vi "Intake Loop.vi"   [LabVIEW 2017]
uses:
  <vilib>/Rock Robotics/WPI/ThirdParty/Phoenix-LabVIEW/Motor Controller/Controls/CTRE_Phoenix_MotorControl_ControlMode.ctl
  <vilib>/Rock Robotics/WPI/ThirdParty/Phoenix-LabVIEW/Motor Controller/Get/CTRE_Phoenix_MotorController_GetSelectedSensorData.vi
  <vilib>/Rock Robotics/WPI/ThirdParty/Phoenix-LabVIEW/Motor Controller/Get/CTRE_Phoenix_MotorController_GetOutputCurrent_Enhanced.vi
  <vilib>/Rock Robotics/WPI/ThirdParty/Phoenix-LabVIEW/Motor Controller/Get/CTRE_Phoenix_MotorController_GetPulseWidthAll.vi
  <vilib>/Rock Robotics/WPI/ThirdParty/Phoenix-LabVIEW/Motor Controller/Get/CTRE_Phoenix_MotorController_GetVoltage.vi
  <vilib>/Rock Robotics/WPI/ThirdParty/Phoenix-LabVIEW/Motor Controller/Get/CTRE_Phoenix_MotorController_GetGeneralStatus.vi
  <vilib>/Rock Robotics/WPI/ThirdParty/Phoenix-LabVIEW/Motor Controller/Get/CTRE_Phoenix_MotorController_GetTemperature.vi
  Robot Global Data.vi
  <vilib>/Rock Robotics/WPI/Solenoid/Deprecated/WPI_SolenoidSetBool.vi
types:
  T1 = typedef "CTRE_Phoenix_MotorControl_ControlMode.ctl" = u16
  T2 = typedef "Intake Status Cluster.ctl" = cluster{"Intake Mode":T3, "Intake States":T4, "Intake Current Angle":dbl, "Cube In Posession?":bool, "Intake Wrist Up?":bool}
  T3 = typedef "Intake Mode.ctl" = enum16{"Auto", "Semi Auto", "Manual"}
  T4 = typedef "Intake States.ctl" = enum16{"Zero", "Override Angle", "Idle", "Drop Mid", "Drop Low", "Outtake", "Intake"}
  T5 = typedef "Intake Command Cluster.ctl" = cluster{"Intake Mode":T3, "Intake States":T4, "Manual Roller Power":dbl, "Manual Close?":bool, "Manual Lift Power":dbl, "Override Lift?":bool, "Override Angle":dbl}
  T6 = typedef "Dashboard Control Data.ctl" = cluster{"Drivetrain Settings Cluster":T7, "Intake Presets":T9, "Elevator Settings Cluster":T10}
  T7 = typedef "Drivetrain Settings Cluster.ctl" = cluster{"Gyro Steer PID Gains":T8, "Distance Drive PID Gains":T8, "Drive Tolerance":dbl, "Gyro Tolerance":dbl, "Gyro Output":dbl, "Distance Output":dbl, "Y Power Multiplier":dbl, "Turn Power Multiplier":dbl, "Creep Rate":dbl, "Constant Power":bool, "DT Mode Modifier":enum16{"None, Default", "Cube", "Square"}, "Left Encoder Tick Constant":dbl, "Right Encoder Tick Constant":dbl, "Shift Speed":dbl}
  T8 = typedef "PID Gains Cluster.ctl" = cluster{"Integral Time":dbl, "Proportional Gain":dbl, "Derivative Time":dbl}
  T9 = typedef "Intake Presets.ctl" = cluster{"Idle Angle":dbl, "Mid Angle":dbl, "Low Angle":dbl, "Outtake Power":dbl, "Intake Power":dbl, "Unstuck":dbl, "Angle Tolerance":dbl, "Max Angle":dbl, "Max Current":dbl, "Current Trip Time":dbl, "Reset Encoder?":bool, "Encoder Scale":dbl, "PID gains":cluster{"proportional gain (Kc)":dbl, "integral time (Ti, min)":dbl, "derivative time (Td, min)":dbl}, "output range":cluster{"output high":dbl, "output low":dbl}}
  T10 = typedef "Elevator Settings Cluster.ctl" = cluster{"Ground Height":dbl, "Switch Height":dbl, "Scale High Height ":dbl, "Scale Low Height":dbl, "Elevator PID Gains":T11, "Elevator Tolerance":dbl, "Reset Encoders":bool, "Encoder Scale":dbl, "Max Height":dbl, "Mid Height":dbl, "output range":cluster{"output high":dbl, "output low":dbl}}
  T11 = typedef "PID Gains.ctl" = cluster{"proportional gain (Kc)":dbl, "integral time (Ti, min)":dbl, "derivative time (Td, min)":dbl}
  T12 = typedef "WPI_MotorControlDeviceRef.ctl" = cluster{"DeviceStatus":errorcluster, "Type":T13, "PWM":cluster{"PWM Channel":T14, "DeadBand":T15}, "CAN":cluster{"Device Number":u8, "SetOutput VI Ref":variant, "GetOutput VI Ref":variant, "Enable VI Ref":variant, "Disable VI Ref":variant, "Data":variant}, "Invert":bool, "DIO PWM":cluster{"PWM \"Enable\" Channel":T14, "DIOChannel":T16, "PWM Rate":dbl}}
  T13 = typedef "WPI_MotorControlType.ctl" = enum16{"PWM", "CAN", "DIO PWM"}
  T14 = typedef "FPGA_DIOPWMChannel.ctl" = enum8{"PWM 0", "PWM 1", "PWM 2", "PWM 3", "PWM 4", "PWM 5", "PWM 6", "PWM 7", "PWM 8", "PWM 9", "PWM MXP 0", "PWM MXP 1", "PWM MXP 2", "PWM MXP 3", "PWM MXP 4", "PWM MXP 5", "PWM MXP 6", "PWM MXP 7", "PWM MXP 8", "PWM MXP 9", "Invalid"}
  T15 = typedef "WPI_PWMDeadband.ctl" = cluster{"Name":string, "maxPositivePwm":i32, "minPositivePwm":i32, "centerPwm":i32, "maxNegativePwm":i32, "minNegativePwm":i32, "angularRange":u16}
  T16 = typedef "FPGA_DIOChannel.ctl" = enum8{"DIO 0", "DIO 1", "DIO 2", "DIO 3", "DIO 4", "DIO 5", "DIO 6", "DIO 7", "DIO 8", "DIO 9", "DIO MXP 0", "DIO MXP 1", "DIO MXP 2", "DIO MXP 3", "DIO MXP 4", "DIO MXP 5", "DIO MXP 6", "DIO MXP 7", "DIO MXP 8", "DIO MXP 9", "DIO MXP 10", "DIO MXP 11", "DIO MXP 12", "DIO MXP 13", "DIO MXP 14", "DIO MXP 15", "SPI Port CS1", "SPI Port CS2", "SPI Port CS3", "SPI Port MISO", "SPI Port MOSI", "Invalid"}
  T17 = typedef "WPI_SwitchDevRef.ctl" = cluster{"DevStatus":errorcluster, "DIO Channel":T16, "CntIndex":T18, "Normally Closed":bool}
  T18 = typedef "FPGA_CounterCtrSystemIndex.ctl" = enum8{"Ctr 0", "Ctr 1", "Ctr 2", "Ctr 3", "Ctr 4", "Ctr 5", "Ctr 6", "Ctr 7", "Invalid"}
  T19 = typedef "WPI_SolenoidDevRef.ctl" = cluster{"DevStatus":errorcluster, "Pneumatics Control Module":u8, "Forward Solenoid Channel":T20, "Reverse Solenoid Channel":T20}
  T20 = typedef "WPI_SolenoidChannel.ctl" = enum8{"Solenoid 0", "Solenoid 1", "Solenoid 2", "Solenoid 3", "Solenoid 4", "Solenoid 5", "Solenoid 6", "Solenoid 7", "Invalid"}
  T21 = typedef "Intake PDP Info.ctl" = cluster{"Voltage Percent Output":dbl, "Output Voltage":dbl, "Bus Voltage":dbl, "Device ID":dbl, "Output Current":dbl, "Sensor Velocity":dbl, "Sensor Position":dbl, "Pulse Width Position":dbl, "Pulse Width Velocity":dbl, "Temperature":dbl, "Inverted?":bool}
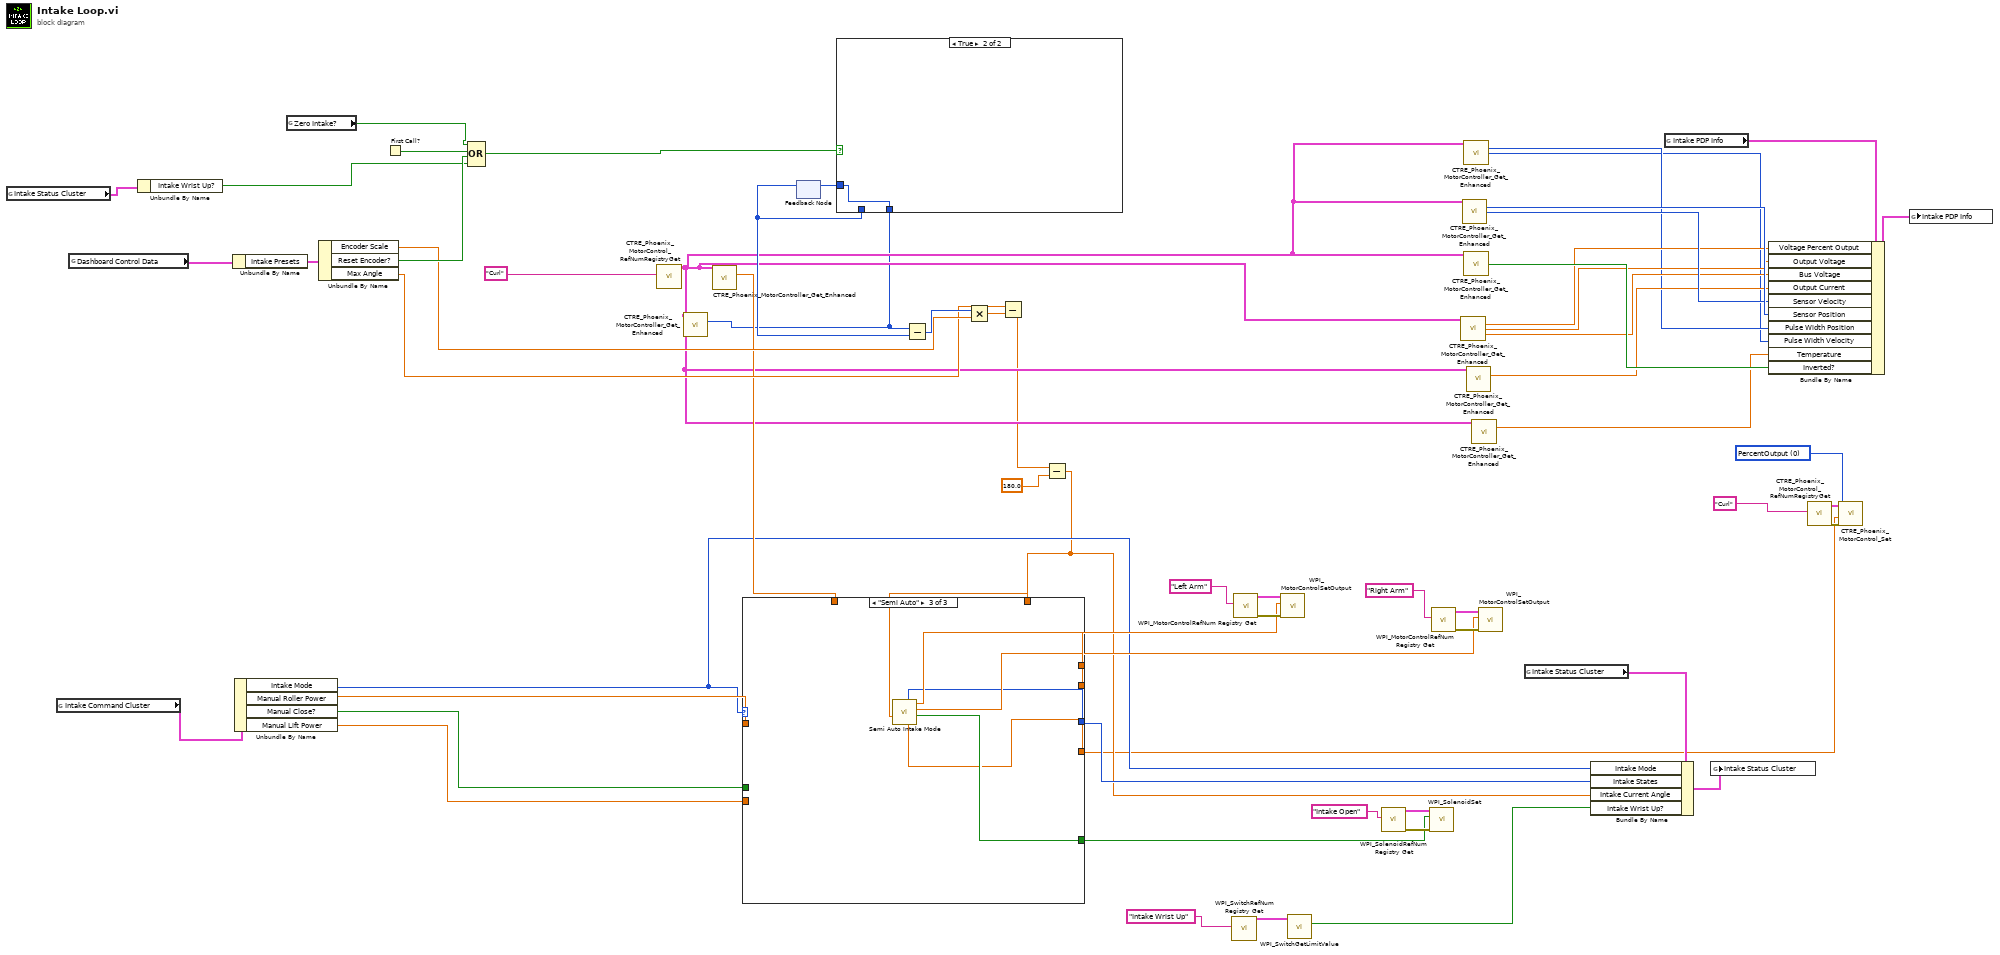
[diagram p0: block diagram]
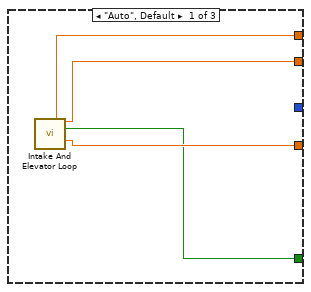
[diagram p2: hidden frame]
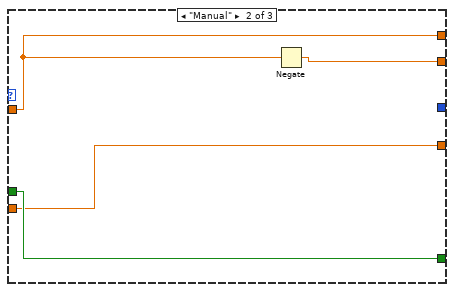
[diagram p3: hidden frame]
diagram:
  w25 = T1 0 items=["PercentOutput"=0, "Position"=1, "Velocity"=2, "Current"=3, "Follower"=5, "MotionProfile"=6, "MotionMagic"=7, "MotionMagicArc"=8, "MotionProfileArc"=10, "Disabled"=15] ("Control Mode")
  n1 = global read "Robot Global Data.vi" "Intake Status Cluster"() -> (w4:T2)
  n2 = global read "Robot Global Data.vi" "Intake Command Cluster"() -> (w52:T5)
  n3 = global read "Robot Global Data.vi" "Dashboard Control Data"() -> (w51:T6)
  n4 = Unbundle By Name(w4) -> ("Intake Wrist Up?"=w3:bool)
  n5 = Unbundle By Name(w51) -> ("Intake Presets"=w50:T9)
  n6 = Unbundle By Name(w52) -> ("Intake Mode"=w10:T3, "Manual Roller Power"=w34:dbl, "Manual Close?"=w33:bool, "Manual Lift Power"=w32:dbl)
  n7 = global read "Robot Global Data.vi" "Zero Intake?"() -> (w47:bool)
  n8 = Unbundle By Name(w50) -> ("Encoder Scale"=w42:dbl, "Reset Encoder?"=w48:bool, "Max Angle"=w40:dbl)
  n9 = First Call?() -> (First Call?: T/F=w49:bool)
  n10 = Compound Arithmetic op=OR(w47, w49, w48, w3) -> (w46:bool)
  n11 = call <vilib>:"CTRE_Phoenix_MotorControl_RefNumRegistryGet.vi"("refnum name"="Curl") -> ("PhoenixMotorControlDevRef"=w19:T12)  [unwired: 9 in, 1 out]
  n12 = call-poly <vilib>:"CTRE_Phoenix_MotorController_Get_Enhanced.vi"("PhoenixMotorControlDevRef"=w19) -> ("Position (Raw Sensor Units)"=w18:i32)  [unwired: 11 in, 3 out]
  n13 = call-poly <vilib>:"CTRE_Phoenix_MotorController_Get_Enhanced.vi"("PhoenixMotorControlDevRef"=w19) -> ("Output Current"=w20:dbl)  [unwired: 12 in, 2 out]
  n14 = feedback #1() -> (w44:i32)  [unwired: 1 in]
  n15 = case shown="True" w46 {
    tunnel: [w62 w63] -> w45
    tunnel: w44 -> [w62 _]
    tunnel: w18 -> [_ w63]
    frame False {
    }
    frame True {
    }
  }
  n16 = feedback-in #1(w45) -> ()
  n17 = Subtract(x=w18, y=w44) -> (x-y=w43:i32)
  n18 = Multiply(x=w43, y=w42) -> (x*y=w41:dbl)
  n19 = Subtract(x=w40, y=w41) -> (x-y=w9:dbl)
  n20 = Subtract(x=w9, y=180.0) -> (x-y=w7:dbl)
  n21 = case shown="\"Semi Auto\"" w10 {
    tunnel: w20 -> [_ _ _]
    tunnel: w7 -> [_ _ w77]
    tunnel: [w67 w69 w76] -> w37
    tunnel: [w66 w70 w75] -> w36
    tunnel: [w65 w68 w73] -> w1
    tunnel: [w64 w71 w74] -> w35
    tunnel: w34 -> [_ w69 _]
    tunnel: w33 -> [_ w71 _]
    tunnel: w32 -> [_ w68 _]
    tunnel: [_ _ w72] -> w31
    frame "Auto", Default {
      n22 = call "Intake And Elevator Loop.vi"() -> ("Intake Left Power"=w67:dbl, "Intake Right Power"=w66:dbl, "Intake Open"=w64:bool, "Intake Angle"=w65:dbl)  [unwired: 11 in, 1 out]
    }
    frame "Manual" {
      n23 = Negate(x=w69) -> (-x=w70:dbl)
    }
    frame "Semi Auto" {
      n24 = call "Semi Auto Intake Mode.vi"("Current Intake Angle"=w77) -> ("Intake Open"=w74:bool, "Intake Right Power"=w75:dbl, "Intake Left Power"=w76:dbl, "Intake Angle"=w73:dbl, "Intake States"=w72:T4)  [unwired: 6 in]
    }
  }
  n25 = call <vilib>:"WPI_SwitchRefNum Registry Get.vi"("refnum name"="Intake Wrist Up") -> ("SwitchDevRef"=w6:T17)  [unwired: 9 in, 1 out]
  n26 = call <vilib>:"WPI_MotorControlRefNum Registry Get.vi"("refnum name"="Left Arm") -> ("error out"=w61:errorcluster, "MotorControlDevRef"=w60:T12)  [unwired: 9 in]
  n27 = call <vilib>:"WPI_MotorControlSetOutput.vi"("error in (no error)"=w61, "Output"=w37, "MotorControlDevRef"=w60) -> ()  [unwired: 6 in, 3 out]
  n28 = call <vilib>:"WPI_SwitchGetLimitValue.vi"("SwitchDevRef"=w6) -> ("Switch Pressed"=w2:bool)  [unwired: 8 in, 2 out]
  n29 = call <vilib>:"WPI_SolenoidRefNum Registry Get.vi"("refnum name"="Intake Open") -> ("error out"=w55:errorcluster, "SolenoidDevRef"=w54:T19)  [unwired: 9 in]
  n30 = call-poly <vilib>:"WPI_SolenoidSet.vi"("error in (no error)"=w55, "Value"=w35, "SolenoidDevRef"=w54) -> ()  [unwired: 7 in, 2 out]
  n31 = call <vilib>:"WPI_MotorControlRefNum Registry Get.vi"("refnum name"="Right Arm") -> ("error out"=w56:errorcluster, "MotorControlDevRef"=w57:T12)  [unwired: 9 in]
  n32 = call-poly <vilib>:"CTRE_Phoenix_MotorController_Get_Enhanced.vi"("PhoenixMotorControlDevRef"=w19) -> ("Percent Output"=w16:dbl, "Output Voltage"=w13:dbl, "Bus Voltage"=w14:dbl)  [unwired: 10 in, 2 out]
  n33 = call-poly <vilib>:"CTRE_Phoenix_MotorController_Get_Enhanced.vi"("PhoenixMotorControlDevRef"=w19) -> ("Position (Raw Sensor Units)"=w23:i32, "Velocity (Raw Sensor Units per 100 ms)"=w17:i32)  [unwired: 11 in, 2 out]
  n34 = call-poly <vilib>:"CTRE_Phoenix_MotorController_Get_Enhanced.vi"("PhoenixMotorControlDevRef"=w19) -> ("Pulse Width Position"=w12:i32, "Pulse Width Velocity"=w11:i32)  [unwired: 9 in, 4 out]
  n35 = call-poly <vilib>:"CTRE_Phoenix_MotorController_Get_Enhanced.vi"("PhoenixMotorControlDevRef"=w19) -> ("Inverted?"=w22:bool)  [unwired: 9 in, 5 out]
  n36 = call-poly <vilib>:"CTRE_Phoenix_MotorController_Get_Enhanced.vi"("PhoenixMotorControlDevRef"=w19) -> ("Output Current"=w15:dbl)  [unwired: 12 in, 2 out]
  n37 = call-poly <vilib>:"CTRE_Phoenix_MotorController_Get_Enhanced.vi"("PhoenixMotorControlDevRef"=w19) -> ("Temperature (C)"=w21:dbl)  [unwired: 12 in, 2 out]
  n38 = call <vilib>:"WPI_MotorControlSetOutput.vi"("error in (no error)"=w56, "Output"=w36, "MotorControlDevRef"=w57) -> ()  [unwired: 6 in, 3 out]
  n39 = global read "Robot Global Data.vi" "Intake Status Cluster"() -> (w39:T2)
  n40 = Bundle By Name(cluster=w39, "Intake Mode"=w10, "Intake States"=w31, "Intake Current Angle"=w7, "Intake Wrist Up?"=w2) -> (w38:T2)
  n41 = global read "Robot Global Data.vi" "Intake PDP Info"() -> (w29:T21)
  n42 = global write "Robot Global Data.vi" "Intake Status Cluster"(w38) -> ()
  n43 = Bundle By Name(cluster=w29, "Voltage Percent Output"=w16, "Output Voltage"=w13, "Bus Voltage"=w14, "Output Current"=w15, "Sensor Velocity"=w17, "Sensor Position"=w23, "Pulse Width Position"=w12, "Pulse Width Velocity"=w11, "Temperature"=w21, "Inverted?"=w22) -> (w28:T21)
  n44 = call <vilib>:"CTRE_Phoenix_MotorControl_RefNumRegistryGet.vi"("refnum name"="Curl") -> ("error out"=w27:errorcluster, "PhoenixMotorControlDevRef"=w26:T12)  [unwired: 9 in]
  n45 = call <vilib>:"CTRE_Phoenix_MotorControl_Set.vi"("error in (no error)"=w27, "Output"=w1, "Control Mode"=w25, "PhoenixMotorControlDevRef"=w26) -> ()  [unwired: 6 in, 2 out]
  n46 = global write "Robot Global Data.vi" "Intake PDP Info"(w28) -> ()
